vi "Get Foreground Wnd Hwnd.vi"(8 "error in (no error)":errorcluster) -> (0 "error out":errorcluster, 3 "hwnd":u32)   [LabVIEW 2019, in "LV MDI.lvclass"]
uses:
  LV MDI.lvclass
  user32.dll
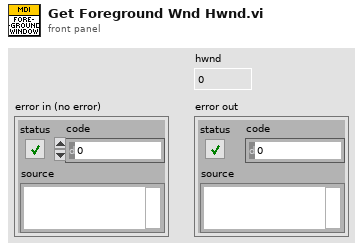
[diagram p1: front panel]
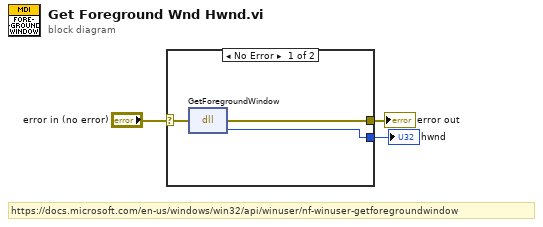
[diagram p0: block diagram]
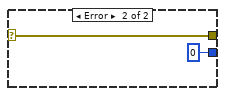
[diagram p2: hidden frame]
diagram:
  # "https://docs.microsoft.com/en-us/windows/win32/api/winuser/nf-winuser-getforegroundwindow"
  n1 = case shown="No Error" "error in (no error)" {
    selector: "error in (no error)" -> [w4 w8]
    tunnel: [w6 u32 0 ("hwnd")] -> w3
    tunnel: [w5 w8] -> w2
    frame No Error {
      n2 = dll-call lib="user32.dll" fn="GetForegroundWindow"(error in=w4) -> (error out=w5:errorcluster, "hwnd"=w6:u32)  [unwired: 2 in, 1 out]
    }
    frame Error {
    }
  }
  "hwnd" <- w3
  "error out" <- w2
